vi "INITIALIZE State Queue.vi"() -> (1 "State que out":T1[](array[typedef]))   [LabVIEW 2011]
uses:
  STATE cluster.ctl
  State Machine Lib.lvlib
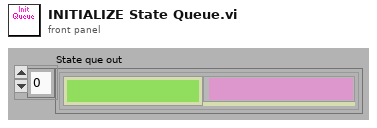
[diagram p1: front panel]
types:
  T1 = typedef "State Machine Lib.lvlib/STATE cluster.ctl" = cluster{"State":string, "Parameters":variant}
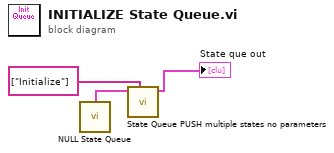
[diagram p0: block diagram]
diagram:
  n1 = call "NULL State Queue.vi"() -> ("NULL State Queue"=w2:T1[])
  n2 = call "State Queue PUSH multiple states no parameters.vi"("States to queue"=string[] ["Initialize"] ("State que in"), "State que in"=w2) -> ("State que out"=→"State que out":T1[])  [unwired: 8 in, 1 out]
